vi "arithmetic.vi"() -> ()   [LabVIEW 2024]
panel:
  out "Numeric 6":dbl
  out "Numeric 5":dbl
  out "Numeric 4":dbl
  out "Numeric 3":dbl
  in  "Numeric 2":dbl
  in  "Numeric":dbl
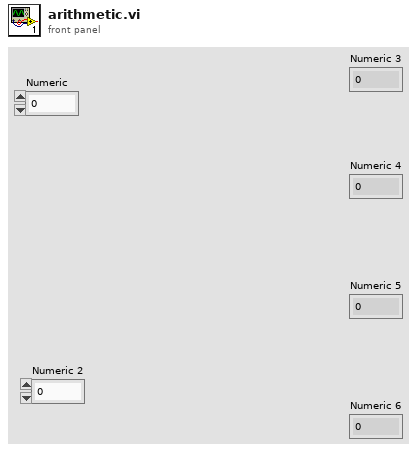
[diagram p1: front panel]
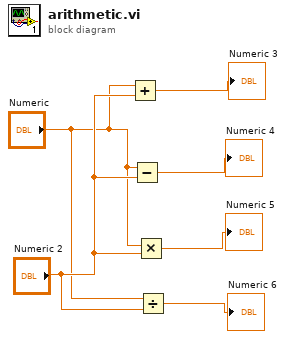
[diagram p0: block diagram]
diagram:
  n1 = Add(x="Numeric", y="Numeric 2") -> (x+y=→"Numeric 3":dbl)
  n2 = Subtract(x="Numeric", y="Numeric 2") -> (x-y=→"Numeric 4":dbl)
  n3 = Multiply(x="Numeric", y="Numeric 2") -> (x*y=→"Numeric 5":dbl)
  n4 = Divide(x="Numeric", y="Numeric 2") -> (x/y=→"Numeric 6":dbl)
